vi "RT LED Module.vi"(4 "LED 3":T4 {"Brightness" max=1000}, 5 "LED 1":T2 {"Brightness" max=1000}, 6 "LED 2":T1 {"Brightness" max=1000}, 7 "LED 0":T3 {"Brightness" max=1000}, 8 "error in":errorcluster, 11 "FPGA VI Reference In":refnum<k20>) -> (0 "error out":errorcluster, 3 "FPGA VI Reference Out":refnum<k20>)   [LabVIEW 2015]
uses:
  <vilib>/Utility/error.llb/Error Cluster From Error Code.vi
  <vilib>/rvi/errors/niLvFpgaAdjustHostInterfaceError.vi
  <vilib>/rvi/interface/nirviReadWriteControl/nirviReadWriteControl.xnode
  NiFpgaLv.dll
  <vilib>/rvi/interface/Simulation/niFpgaSimulationCallBeginRW.vi
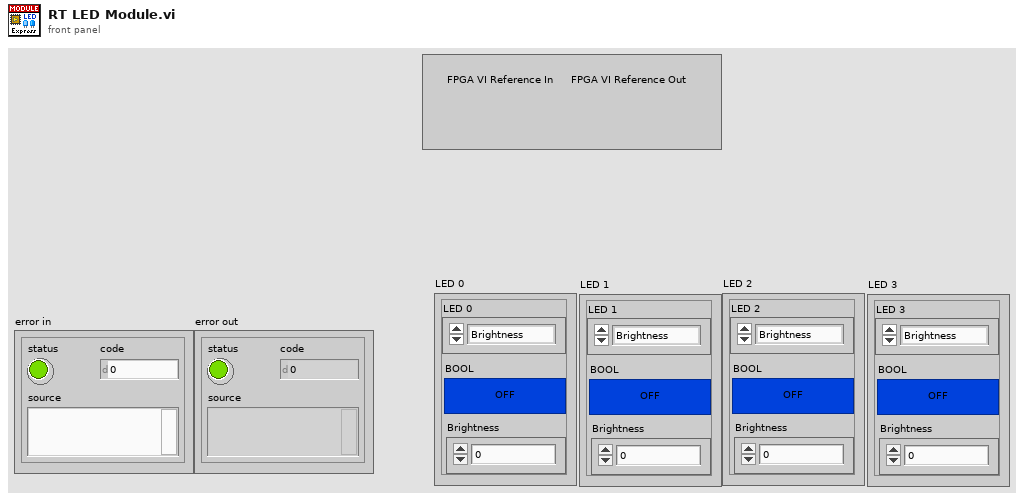
[diagram p1: front panel]
types:
  T1 = cluster{"LED 2":enum16{"Brightness", "Bool"}, "BOOL":bool, "Brightness":u32}
  T2 = cluster{"LED 1":enum16{"Brightness", "Bool"}, "BOOL":bool, "Brightness":u32}
  T3 = cluster{"LED 0":enum16{"Brightness", "Bool"}, "BOOL":bool, "Brightness":u32}
  T4 = cluster{"LED 3":enum16{"Brightness", "Bool"}, "BOOL":bool, "Brightness":u32}
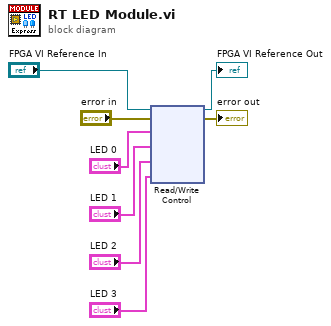
[diagram p0: block diagram]
diagram:
  n1 = xnode "Read/Write Control"("FPGA VI Reference In"="FPGA VI Reference In", "error in"="error in", "LED 0"="LED 0", "LED 1"="LED 1", "LED 2"="LED 2", "LED 3"="LED 3") -> ("FPGA VI Reference Out"=→"FPGA VI Reference Out":refnum<k20>, "error out"=→"error out":errorcluster)
